vi "Perform Auto-Calibration.vi"(8 "error in (no error)":errorcluster, 11 "VISA resource name":refnum<visa-resource-name>) -> (0 "error out":errorcluster, 2 "Auto-Cal Passed?":bool, 3 "VISA resource name out":refnum<visa-resource-name>)   [LabVIEW 2018, in "DPO4104.lvlib" / "DPO4104.lvclass"]
doc: "This VI sends the calibration command to the oscilloscope."
uses:
  DPO4104.lvclass
  <instrlib>/Tektronix DPO MSO 2000 4000 Series/Tektronix DPO MSO 2000 4000 Series.lvlib
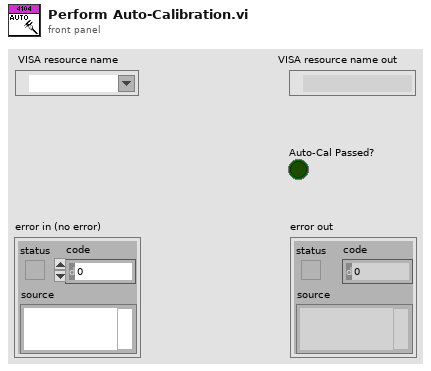
[diagram p1: front panel]
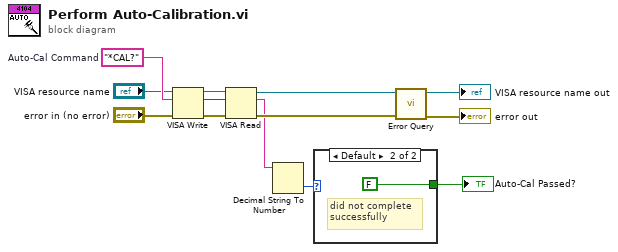
[diagram p0: block diagram]
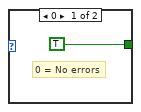
[diagram p2: hidden frame]
diagram:
  w9 = "*CAL?"  # Auto-Cal Command
  n1 = VISA Write(VISA resource name="VISA resource name", write buffer=w9, error in (no error)="error in (no error)") -> (VISA resource name out=w13:refnum<visa-resource-name>, return count=w1:u32, error out=w12:errorcluster)
  n2 = VISA Read(VISA resource name=w13, byte count=w1, error in (no error)=w12) -> (VISA resource name out=w5:refnum<visa-resource-name>, read buffer=w3:string, error out=w6:errorcluster)  [unwired: 1 out]
  n3 = Decimal String To Number(string=w3) -> (number=w4:i32)  [unwired: 2 in, 1 out]
  n4 = case shown="Default" w4 {
    tunnel: [TRUE FALSE] -> w2
    frame 0 {
      # "0 = No errors"
    }
    frame Default {
      # "did not complete\nsuccessfully"
    }
  }
  "Auto-Cal Passed?" <- w2
  n5 = call <instrlib>:"Error Query.vi"("error in (no error)"=w6, "VISA resource name"=w5) -> ("error out"=→"error out":errorcluster, "VISA resource name out"=→"VISA resource name out":refnum<visa-resource-name>)  [unwired: 6 in, 2 out]
